vi "Dequeue.vi"(6 "Instance":i32, 10 "Loop Tick":i32=200, 11 "Loop Counter":i32) -> (0 "error out":errorcluster, 1 "ResponseNotifcation":refnum<notifier>, 2 "Data":variant, 3 "Msg":string, 4 "Exit?":bool)   [LabVIEW 2017, in "Communication.lvlib"]
uses:
  Communication.lvlib
  QueueRepo.Action.ctl
  MsgData.ctl
  MsgAck.ctl
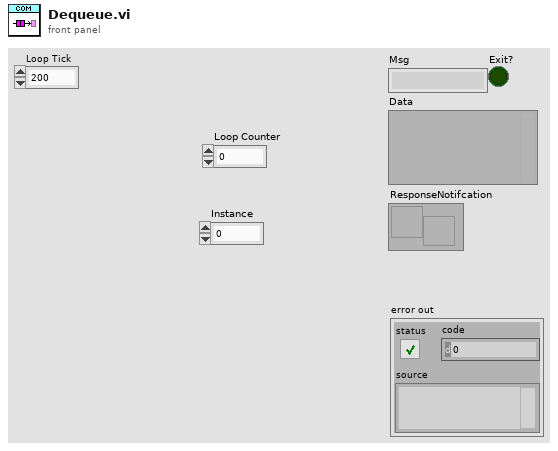
[diagram p1: front panel]
types:
  T1 = typedef "Communication.lvlib/QueueRepo.Action.ctl" = enum16{"Add", "Get", "Destroy", "Get All", "Clear"}
  T2 = typedef "Communication.lvlib/MsgData.ctl" = cluster{"Msg":string, "Data":variant, "Ack":refnum<notifier>}
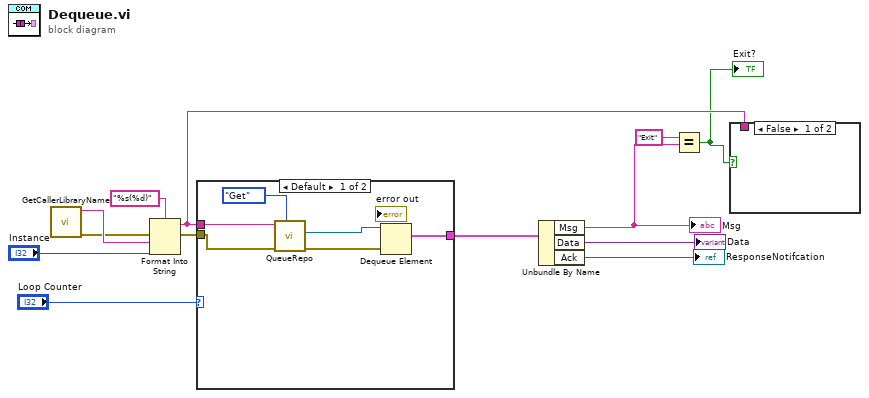
[diagram p0: block diagram]
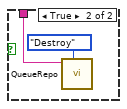
[diagram p2: hidden frame]
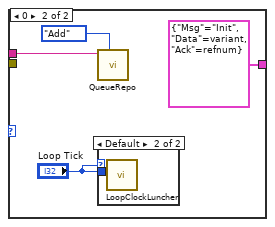
[diagram p3: hidden frame]
diagram:
  n1 = call "GetCallerLibraryName.vi"() -> ("error out"=w9:errorcluster, "Name"=w10:string)  [unwired: 10 in]
  n2 = Format Into String(format string="%s(%d)", error in=w9, w10, "Instance") -> (resulting string=w2:string, error out=w8:errorcluster)  [unwired: 1 in]
  n3 = case shown="Default" "Loop Counter" {
    tunnel: w2 -> [w18 w23]
    tunnel: w8 -> [w17 _]
    tunnel: [w14 T2 {"Msg"="Init", "Data"=variant, "Ack"=refnum} ("Cluster")] -> w7
    frame Default {
      n4 = call "QueueRepo.vi"("Action"=QueueRepo.Action."Get", "error in (no error)"=w17, "Name"=w18) -> ("error out"=w16:errorcluster, "queue out"=w15:refnum<queue>)  [unwired: 5 in, 2 out]
      n5 = Dequeue Element(queue=w15, error in (no error)=w16) -> (element=w14:T2)  [unwired: 1 in, 3 out]
    }
    frame 0 {
      n6 = call "QueueRepo.vi"("Action"=QueueRepo.Action."Add", "Name"=w23) -> ()  [unwired: 6 in, 4 out]
      n7 = case shown="Default" "Loop Tick" {
        tunnel: "Loop Tick" -> [_ w24]
        frame -1 {
        }
        frame Default {
          n8 = call "LoopClockLuncher.vi"("milliseconds to wait"=w24) -> ()  [unwired: 9 in, 2 out]
        }
      }
    }
  }
  n9 = Unbundle By Name(w7) -> ("Msg"=w4:string, "Data"=→"Data":variant, "Ack"=→"ResponseNotifcation":refnum<notifier>)
  "Msg" <- w4
  n10 = Equal?(x="Exit", y=w4) -> (x = y?=w1:bool)
  "Exit?" <- w1
  n11 = case shown="False" w1 {
    tunnel: w2 -> [_ w26]
    frame False {
    }
    frame True {
      n12 = call "QueueRepo.vi"("Action"=QueueRepo.Action."Destroy", "Name"=w26) -> ()  [unwired: 6 in, 4 out]
    }
  }
